vi "Configure Trigger (Ethernet - IP Header).vi"(0 "VISA resource name":refnum<visa-resource-name>, 1 "Protocol (\"XXXXXXXX\")":string="XXXXXXXX", 5 "Trigger Source (9: Bus 1)":u16(ring)=9 items=["Bus 1"=9, "Bus 2"=10], 7 "Source Address (\"XXXXXXXX\")":string="XXXXXXXX", 9 "Destination Address (\"XXXXXXXX\")":string="XXXXXXXX", 11 "error in (no error)":errorcluster) -> (4 "VISA resource name out":refnum<visa-resource-name>, 15 "error out":errorcluster)   [LabVIEW 2009, in "Tektronix DPO MSO 2000 4000 Series.lvlib"]
doc: "Configures IP header trigger settings for Ethernet trigger. \n\n<B>Note:</B>\nThis VI only applies to DPO4034B, DPO4054B, DPO4104B, MSO4034B, MSO4054B, MSO4104B."
uses:
  <instrlib>/Tektronix DPO MSO 2000 4000 Series/Tektronix DPO MSO 2000 4000 Series.lvlib
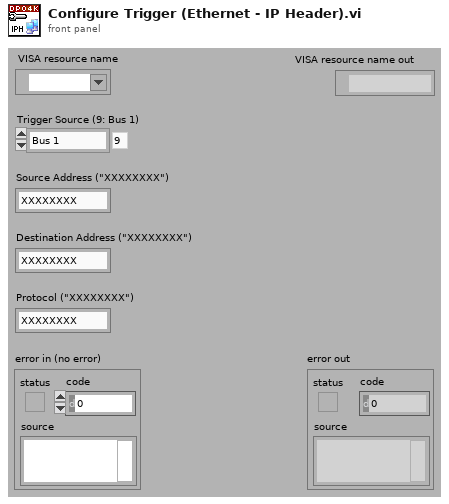
[diagram p1: front panel]
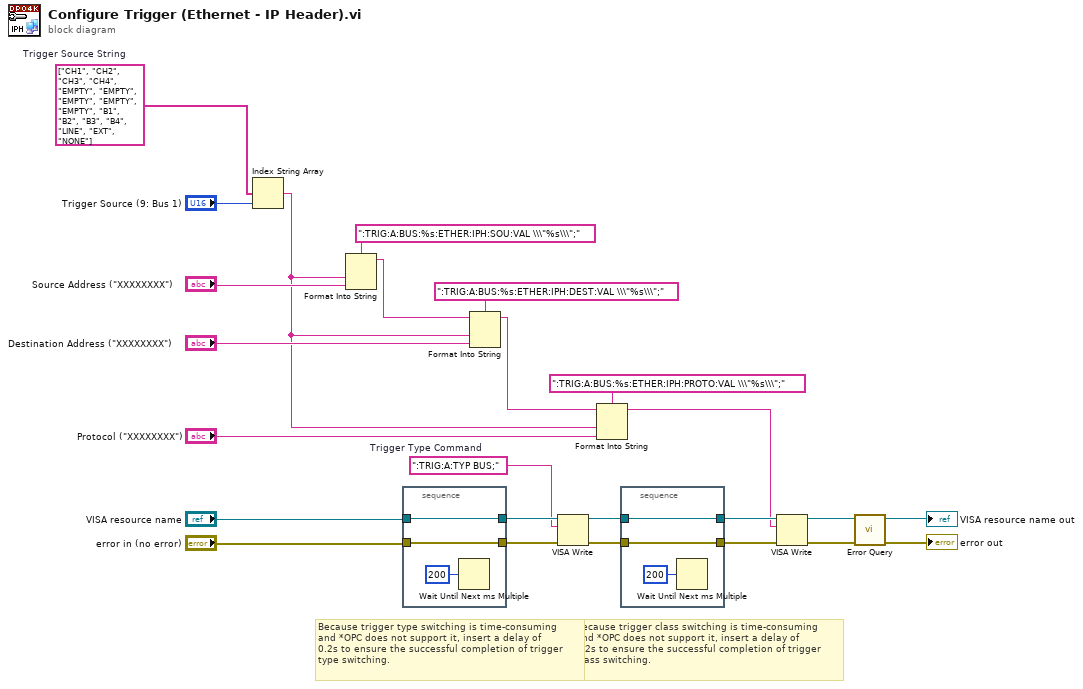
[diagram p0: block diagram]
diagram:
  w18 = string[] ["CH1", "CH2", "CH3", "CH4", "EMPTY", "EMPTY", "EMPTY", "EMPTY", "EMPTY", "B1", "B2", "B3", "B4", "LINE", "EXT", "NONE"]  # Trigger Source String
  w23 = ":TRIG:A:TYP BUS;"  # Trigger Type Command
  # "Because trigger class switching is time-consuming\nand *OPC does not support it, insert a delay of\n0.2s to ensure the successful completion of trigger\nclass switching."
  # "Because trigger type switching is time-consuming\nand *OPC does not support it, insert a delay of\n0.2s to ensure the successful completion of trigger\ntype switching."
  n1 = Index String Array(1:"Trigger Source (9: Bus 1)", 2:w18) -> (0:w2:string)  [unwired: 1 in]
  n2 = Format Into String(format string=":TRIG:A:BUS:%s:ETHER:IPH:SOU:VAL \\\"%s\\\";", w2, "Source Address (\"XXXXXXXX\")") -> (resulting string=w6:string)  [unwired: 2 in, 1 out]
  n3 = stacked-sequence {
    tunnel: "VISA resource name" -> [w27]
    tunnel: [w27] -> w25
    tunnel: "error in (no error)" -> [w26]
    tunnel: [w26] -> w24
    frame #0 {
      n4 = Wait Until Next ms Multiple(millisecond multiple=u32 200) -> ()  [unwired: 1 out]
    }
  }
  n5 = Format Into String(format string=":TRIG:A:BUS:%s:ETHER:IPH:DEST:VAL \\\"%s\\\";", initial string=w6, w2, "Destination Address (\"XXXXXXXX\")") -> (resulting string=w3:string)  [unwired: 1 in, 1 out]
  n6 = VISA Write(VISA resource name=w25, write buffer=w23, error in (no error)=w24) -> (VISA resource name out=w22:refnum<visa-resource-name>, error out=w21:errorcluster)  [unwired: 1 out]
  n7 = Format Into String(format string=":TRIG:A:BUS:%s:ETHER:IPH:PROTO:VAL \\\"%s\\\";", initial string=w3, w2, "Protocol (\"XXXXXXXX\")") -> (resulting string=w1:string)  [unwired: 1 in, 1 out]
  n8 = stacked-sequence {
    tunnel: w22 -> [w30]
    tunnel: [w30] -> w20
    tunnel: w21 -> [w29]
    tunnel: [w29] -> w19
    frame #0 {
      n9 = Wait Until Next ms Multiple(millisecond multiple=u32 200) -> ()  [unwired: 1 out]
    }
  }
  n10 = VISA Write(VISA resource name=w20, write buffer=w1, error in (no error)=w19) -> (VISA resource name out=w16:refnum<visa-resource-name>, error out=w15:errorcluster)  [unwired: 1 out]
  n11 = call <instrlib>:"Error Query.vi"("error in (no error)"=w15, "VISA resource name"=w16) -> ("error out"=→"error out":errorcluster, "VISA resource name out"=→"VISA resource name out":refnum<visa-resource-name>)  [unwired: 6 in, 2 out]
